vi "Initialize Attributes.vi"(8 "error in (no error)":errorcluster, 10 "Attribute Data":variant, 11 "IVI_DMM_Delayed in":refnum<class "IVI_DMM_Delayed.lvclass">) -> (0 "error out":errorcluster, 2 "Found?":bool, 3 "IVI_DMM_Delayed out":refnum<class "IVI_DMM_Delayed.lvclass">)   [LabVIEW 2015, in "IVI_DMM.lvlib" / "IVI_DMM_Delayed.lvclass"]
doc: "Initialize object attribute.\n\nUnique resources should be allocated elsewhere!"
uses:
  IVI_DMM_Delayed.lvclass
  IVI_DMM_Delayed.lvclass/IVI_DMM_Delayed.ctl
  IVI_DMM/IVI_DMM.lvclass
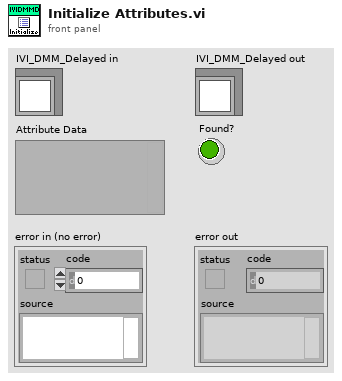
[diagram p1: front panel]
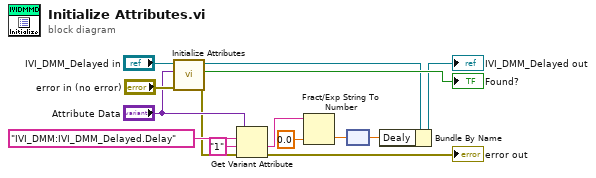
[diagram p0: block diagram]
diagram:
  n1 = call-parent "Initialize Attributes.vi"("error in (no error)"="error in (no error)", "Attribute Data"="Attribute Data", "IVI_DMM in"="IVI_DMM_Delayed in") -> ("error out"=w8:errorcluster, "Found?"=→"Found?":bool, "IVI_DMM out"=w6:refnum<class "IVI_DMM_Delayed.lvclass">)  [unwired: 6 in]
  n2 = Get Variant Attribute(Variant="Attribute Data", name="IVI_DMM:IVI_DMM_Delayed.Delay", default value (empty Variant)="1", error in=w8) -> (value=w4:string, error out=→"error out":errorcluster)  [unwired: 2 out]
  n3 = Fract/Exp String To Number(string=w4, default (0 dbl)=0.0 ("default (0 DBL)")) -> (number=w2:dbl)  [unwired: 2 in, 1 out]
  n4 = node(w2) -> (w1:dbl[unit])
  n5 = Bundle By Name(cluster=w6, "Dealy"=w1) -> (→"IVI_DMM_Delayed out":refnum<class "IVI_DMM_Delayed.lvclass">)
